vi "Configure Measurement.vi"   [LabVIEW 2020, in "Keithley 2000.lvlib"]
doc: "This polymorphic VI configures the mode of the instrument as well as any settings specific to those modes."
uses:
  <instrlib>/Keithley 2000/Keithley 2000.lvlib
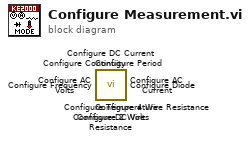
[diagram p0: block diagram]
diagram:
  n1 = call <instrlib>:"Configure Temperature.vi"() -> ()  [unwired: 18 in, 2 out]
  n2 = call <instrlib>:"Configure Period.vi"() -> ()  [unwired: 18 in, 2 out]
  n3 = call <instrlib>:"Configure Frequency.vi"() -> ()  [unwired: 18 in, 2 out]
  n4 = call <instrlib>:"Configure Diode.vi"() -> ()  [unwired: 18 in, 2 out]
  n5 = call <instrlib>:"Configure DC Volts.vi"() -> ()  [unwired: 18 in, 2 out]
  n6 = call <instrlib>:"Configure DC Current.vi"() -> ()  [unwired: 18 in, 2 out]
  n7 = call <instrlib>:"Configure Continuity.vi"() -> ()  [unwired: 18 in, 2 out]
  n8 = call <instrlib>:"Configure AC Volts.vi"() -> ()  [unwired: 18 in, 2 out]
  n9 = call <instrlib>:"Configure AC Current.vi"() -> ()  [unwired: 18 in, 2 out]
  n10 = call <instrlib>:"Configure 4 Wire Resistance.vi"() -> ()  [unwired: 18 in, 2 out]
  n11 = call <instrlib>:"Configure 2 Wire Resistance.vi"() -> ()  [unwired: 18 in, 2 out]
